vi "Send.vi"(2 "string to write":i32(ring) items=["*RST", "*VER", "*CA1", "*CA2", "*SS1", "*SS2", "*SU1", "*SU2", "*SD1", "*SD2", "*CS1", "*CS2", "*AT1", "*AT2", "*AN1", "*AN2", "*PW1", "*PW2", "*TL1", "*TL2", "*ST1", "*ST2", "*ET1", "*ET2", "*EM1", "*EM2", "*SC1", "*SC2"], 3 "error in (no error)":errorcluster, 4 "port number":refnum<visa-resource-name>, 5 "Option":string) -> (0 "error out":errorcluster, 1 "VISA resource name out":refnum<visa-resource-name>)   [LabVIEW 2020]
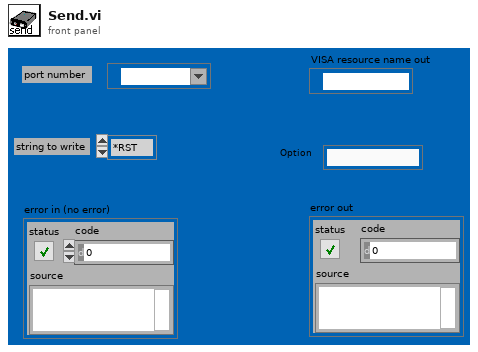
[diagram p1: front panel]
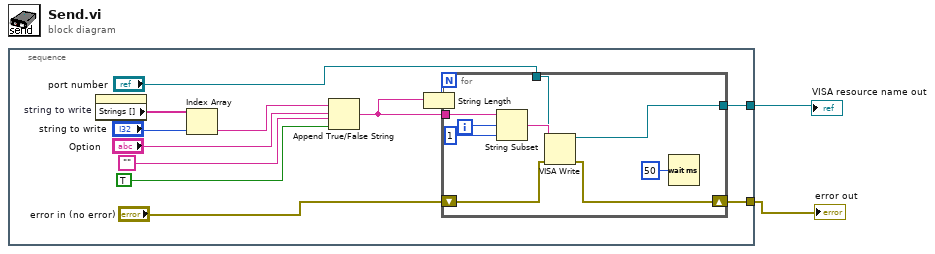
[diagram p0: block diagram]
diagram:
  n1 = stacked-sequence {
    tunnel: [w5] -> w2
    tunnel: [w3] -> w1
    frame #0 {
      n2 = property on="string to write" class="Ring (strict)"() -> ("Strings []"=w13:string[])  [unwired: 2 in, 2 out]
      n3 = Index Array(array=w13, index="string to write") -> (element=w12:string)
      n4 = Append True/False String(1:TRUE ("selector"), 2:"", 3:"Option", 4:w12) -> (0:w6:string)
      n5 = String Length(string=w6) -> (length=w8:i32)
      n6 = for {
        N: w8 -> [_]
        tunnel: w6 -> [w21]
        tunnel: "port number" -> [w18]
        tunnel: [w17] -> w5
        shift-right: [w15] -> w3
        shift-left: "error in (no error)" -> [w16]
        i -> [w22]
        n7 = String Subset(string=w21, offset (0)=w22, length (rest)=1 ("length (rest)")) -> (substring=w19:string)
        n8 = VISA Write(VISA resource name=w18, write buffer=w19, error in (no error)=w16) -> (VISA resource name out=w17:refnum<visa-resource-name>, error out=w15:errorcluster)  [unwired: 1 out]
        n9 = Wait (ms)(milliseconds to wait=u32 50) -> ()  [unwired: 1 out]
      }
    }
  }
  "VISA resource name out" <- w2
  "error out" <- w1
